vi "SPITxWrite.vi"(8 "error in (no error)":errorcluster caption="错误输入（无错误）", 10 "data":u8[](array[numeric]), 11 "handle":u64) -> (0 "error out":errorcluster caption="错误输出", 2 "function return":i32, 3 "handle out":u64)   [LabVIEW 2018]
doc: "Send SPI data"
uses:
  InstrumentsPlayground.lvlib
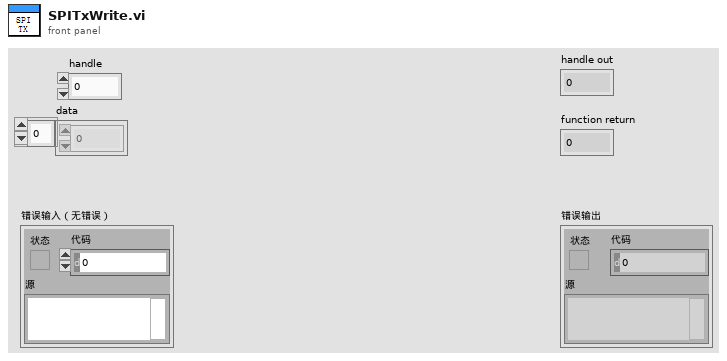
[diagram p1: front panel]
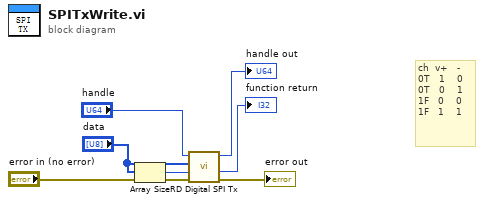
[diagram p0: block diagram]
diagram:
  # "ch  v+   -\n0T   1    0\n0T   0    1\n1F   0    0\n1F   1    1"
  n1 = Array Size(array="data") -> (size(s)=w4:i32)
  n2 = call "RD Digital SPI Tx.vi"("error in (no error)"="error in (no error)", "length"=w4, "data"="data", "handle"="handle") -> ("error out"=→"error out":errorcluster, "function return"=→"function return":i32, "handle out"=→"handle out":u64)  [unwired: 5 in]
